vi "APC_9049_keyKnock.vi"(0 "Knock":bool[](array[boolean])) -> ()   [LabVIEW 2020]
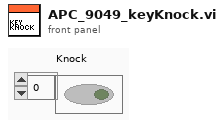
[diagram p1: front panel]
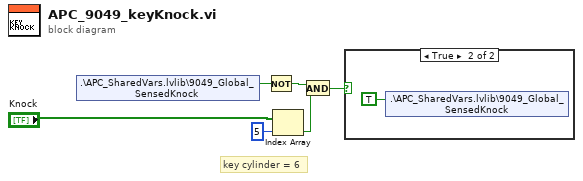
[diagram p0: block diagram]
diagram:
  # "key cylinder = 6"
  n1 = shared-variable ".\\APC_SharedVars.lvlib\\9049_Global_SensedKnock"() -> (w6:bool)  [unwired: 1 in, 1 out]
  n2 = Not(x=w6) -> (.not. x?=w4:bool)
  n3 = Index Array(array="Knock", index=5) -> (element=w3:bool)
  n4 = And(x=w4, y=w3) -> (x .and. y?=w2:bool)
  n5 = case shown="True" w2 {
    frame False {
    }
    frame True {
      n6 = shared-variable ".\\APC_SharedVars.lvlib\\9049_Global_SensedKnock"(TRUE ("9049_Global_SensedKnock")) -> ()  [unwired: 1 in, 1 out]
    }
  }
